vi "SendUpdatePassword.vi"(7 "Device Id":string, 8 "error in (no error)":errorcluster, 9 "New Password":string, 10 "Serial Number":u64 format="%.0x", 11 "Qbus in":refnum<class "Qbus.lvclass">) -> (0 "error out":errorcluster, 3 "Qbus out":refnum<class "Qbus.lvclass">)   [LabVIEW 2017, in "ServerComm.lvlib"]
doc: "Writes the properties the device uses to identify and connect to NI InsightCM Server, as well as to become authorized to come online."
uses:
  <vilib>/addons/InsightCM/Devices/Shared/Common/ServerComm/ServerComm.lvlib
  <vilib>/addons/Qbus/Qbus.lvclass
  <vilib>/addons/InsightCM/Devices/Shared/Common/ServerComm/controls/UpdatePassword.ctl
  <vilib>/addons/InsightCM/Devices/Shared/Ble/BleComm/BleComm.lvlib
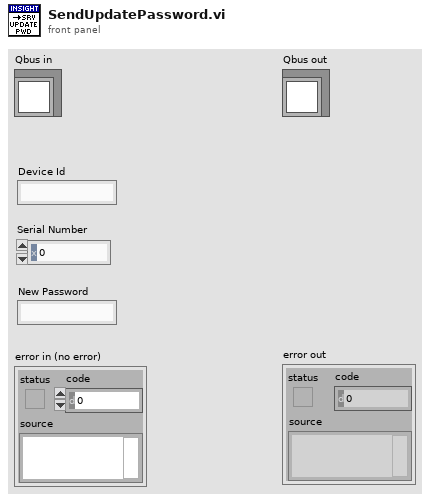
[diagram p1: front panel]
types:
  T1 = typedef "ServerComm.lvlib/UpdatePassword.ctl" = cluster{"Device Id":string, "Serial Number":string, "New Password":string}
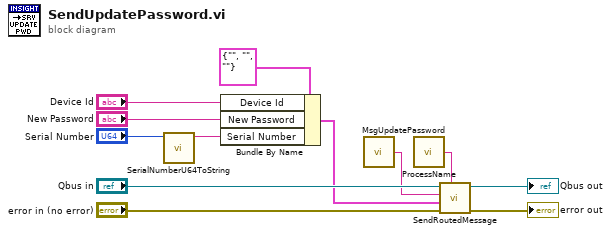
[diagram p0: block diagram]
diagram:
  n1 = call <vilib>:"SerialNumberU64ToString.vi"("serial number u64"="Serial Number") -> ("serial number string"=w2:string)  [unwired: 10 in]
  n2 = Bundle By Name(cluster=T1 {"Device Id"="", "Serial Number"="", "New Password"=""} ("Update Password"), "Device Id"="Device Id", "New Password"="New Password", "Serial Number"=w2) -> (w3:T1)
  n3 = call <vilib>:"MsgUpdatePassword.vi"() -> ("message name"=w7:string)  [unwired: 5 in]
  n4 = call <vilib>:"ProcessName.vi"() -> ("process name"=w9:string)  [unwired: 5 in]
  n5 = call <vilib>:"SendRoutedMessage.vi"("listener process"=w9, "error in (no error)"="error in (no error)", "message value"=w3, "message name"=w7, "Qbus in"="Qbus in") -> ("error in (no error)"=→"error out":errorcluster, "Qbus out"=→"Qbus out":refnum<class "Qbus.lvclass">)  [unwired: 5 in]
